vi "Set configuration chain.vi"(8 "error in (no error)":errorcluster, 9 "class names":string[](array[string]), 10 "configuration":variant[](array[variant]), 11 "Cobolt in":refnum<class "Cobolt.lvclass">) -> (0 "error out":errorcluster, 3 "Cobolt out":refnum<class "Cobolt.lvclass">)   [LabVIEW 2012, in "Cobolt.lvclass"]
uses:
  Cobolt.lvclass
  <vilib>/Distrio/Murmex/Murmex/Murmex.lvclass
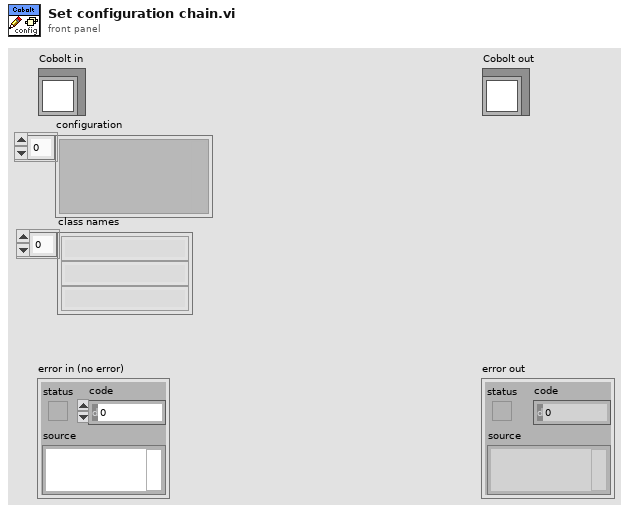
[diagram p1: front panel]
types:
  T1 = typedef "Cobolt.lvclass/configuration_cluster.ctl" = cluster{"VISA resource name":string, "Enable Termination Char":u16, "Baud rate":u32, "data bits":u16, "Flow control":u16, "stop bits":u16, "parity":u16, "Time out":u32, "VISA Wait":dbl[unit], "Laser line":T2, "Generate Error if Fail":bool}
  T2 = typedef "Cobolt.lvclass/laser lines.ctl" = u16
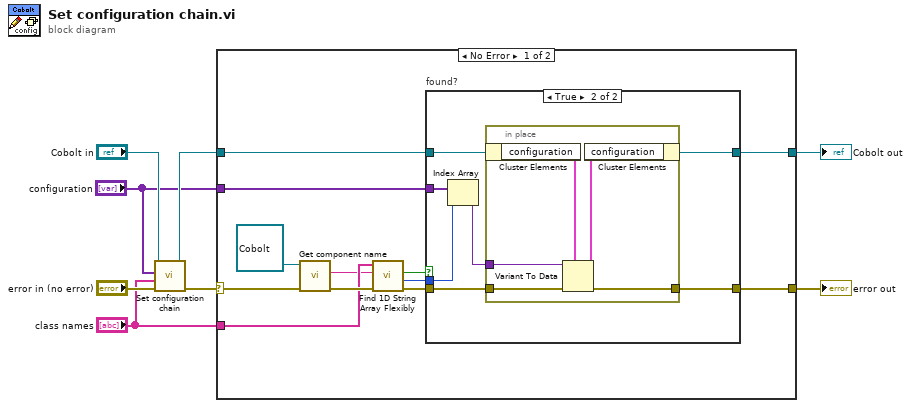
[diagram p0: block diagram]
diagram:
  n1 = call-parent "Set configuration chain.vi"("error in (no error)"="error in (no error)", "class names"="class names", "configuration"="configuration", "Murmex in"="Cobolt in") -> ("error out"=w6:errorcluster, "Murmex out"=w4:refnum<class "Cobolt.lvclass">)  [unwired: 6 in]
  n2 = case shown="No Error" w6 {
    selector: w6 -> [w20 w36]
    tunnel: [w12 w36] -> w5
    tunnel: w4 -> [w10 w35]
    tunnel: [w11 w35] -> w3
    tunnel: "configuration" -> [w9 _]
    tunnel: "class names" -> [w17 _]
    frame No Error {
      n3 = call <vilib>:"Get component name.vi"("error in (no error)"=w20, "Murmex in"=refnum<class "Cobolt.lvclass"> refnum ("Cobolt in")) -> ("error out"=w18:errorcluster, "component name"=w16:string)  [unwired: 7 in, 1 out]
      n4 = call <vilib>:"Find 1D String Array Flexibly.vi"("error in (no error)"=w18, "element"=w16, "array"=w17) -> ("error out"=w13:errorcluster, "index of element"=w14:i32, "found?"=w15:bool)  [unwired: 6 in]
      n5 = case "found?" shown="True" w15 {
        tunnel: w14 -> [_ w27]
        tunnel: w13 -> [w22 w26]
        tunnel: [w22 w25] -> w12
        tunnel: [w21 w23] -> w11
        tunnel: w10 -> [w21 w29]
        tunnel: w9 -> [_ w28]
        frame False {
        }
        frame True {
          n6 = Index Array(array=w28, index=w27) -> (element=w24:variant)
          n7 = in-place {
            in-place-border: w26 -> [w34]
            in-place-border: [w33] -> w25
            in-place-border: w24 -> [w30]
            n8 = in-place-cluster #1(w29) -> ("configuration"=w32:T1)
            n9 = Variant To Data(error in=w34, type=w32, Variant=w30) -> (data=w31:T1, error out=w33:errorcluster)
            n10 = in-place-cluster #1("configuration"=w31) -> (w23:refnum<class "Cobolt.lvclass">)
          }
        }
      }
    }
    frame Error {
    }
  }
  "error out" <- w5
  "Cobolt out" <- w3
